vi "Read Config.vi"() -> (0 "error out":errorcluster)   [LabVIEW 2009]
panel:
  in  "Names":string[](array[string])=["PRODUCT_ID", "HARDWARE_VERSION", "FIRMWARE_VERSION", "BOOTLOADER_VERSION", "WIFI_VERSION", "SERIAL_NUMBER", "POWER_ETHERNET_DEFAULT", "POWER_WIFI_DEFAULT", "POWER_AIN_DEFAULT", "POWER_LED_DEFAULT"]
  out "Error String":string="No Error"
  out "ConnectionType Out":i32=4
  out "DeviceType Out":i32=7
  in  "Identifier":string="10.251.235.236"
  in  "ConnectionType":string="WIFI"
  in  "DeviceType":string="LJM_dtANY"
  in  "NumFrames":i32=10
  out "Values":dbl[](array[numeric])=[7.0, 1.2999999523162842, 1.0118999481201172, 0.9399999976158142, 3.119999885559082, 470010806.0, 1.0, 1.0, 1.0, 1.0] format="%.4f"
  out "Error Frame":i32
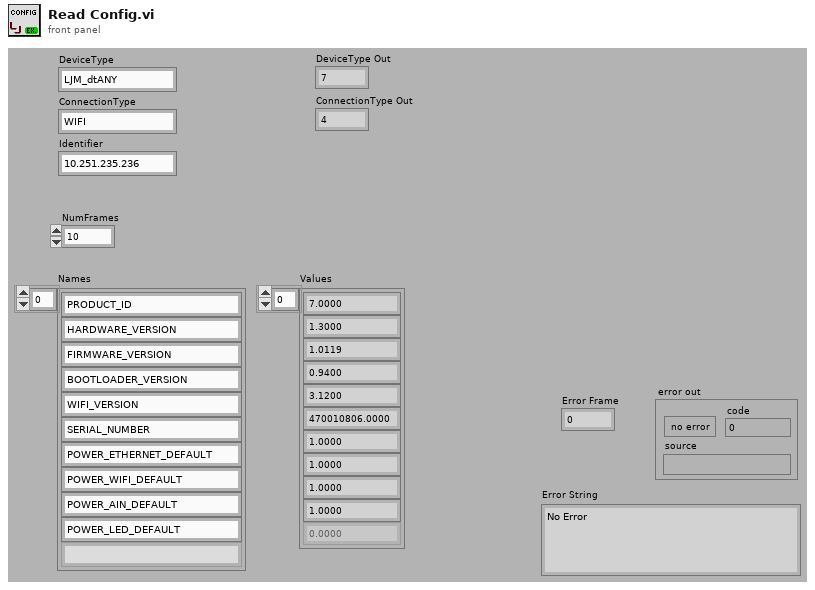
[diagram p1: front panel]
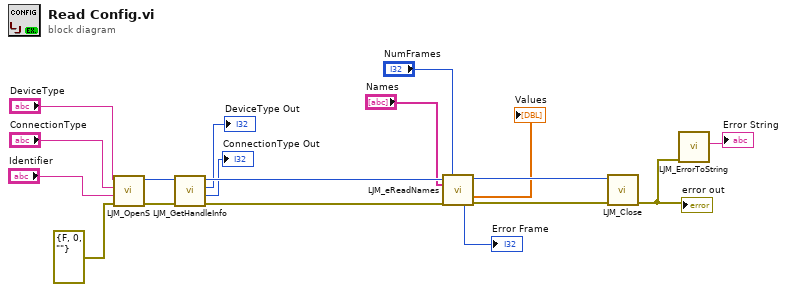
[diagram p0: block diagram]
diagram:
  n1 = call <vilib>:"LJM_OpenS.vi"("error in"=errorcluster {"status"=FALSE, "code"=0, "source"=""} ("error in (no error)"), "Identifier"="Identifier", "ConnectionType"="ConnectionType", "DeviceType"="DeviceType") -> ("error out"=w15:errorcluster, "Handle"=w13:i32)  [unwired: 6 in]
  n2 = call <vilib>:"LJM_GetHandleInfo.vi"("error in"=w15, "Handle In"=w13) -> ("error out"=w14:errorcluster, "ConnectionType"=→"ConnectionType Out":i32, "DeviceType"=→"DeviceType Out":i32, "Handle Out"=w12:i32)  [unwired: 2 in, 4 out]
  n3 = call <vilib>:"LJM_eReadNames.vi"("Handle In"=w12, "NumFrames"="NumFrames", "aNames"="Names", "error in"=w14) -> ("Handle Out"=w11:i32, "aValuesOut"=→"Values":dbl[], "ErrorAddress"=→"Error Frame":i32, "error out"=w17:errorcluster)  [unwired: 8 in]
  n4 = call <vilib>:"LJM_Close.vi"("error in"=w17, "Handle"=w11) -> ("error out"=w5:errorcluster)  [unwired: 9 in]
  "error out" <- w5
  n5 = call <vilib>:"LJM_ErrorToString.vi"("error in"=w5) -> ("String"=→"Error String":string)  [unwired: 10 in]
